vi "ImgLnExp.vi"(7 "Ln/Exp(Ln)":bool, 8 "EorIn":errorcluster, 10 "Dst":T1(plugin-control), 11 "Src":T1(plugin-control)) -> (0 "ErrOut":errorcluster, 3 "ImgOut":T1(plugin-control))   [LabVIEW 2014]
doc: "Use this template to build a VI to use as a subVI."
panel:
  out "size(s)":i32[](array[numeric])
  out "Image Pixels (Float)":sgl[][](array[numeric]) format="%.2f"
  # "Output Parameters"
  # "Input Parameters"
  # "VI Description:\nThis VI is .."
  # ":: MVi Framework V1.0 ::\nAuthor:Gaoke Yang\nEmail: gaoke.yang@yahoo.com\nWeb: www.mvicontrol.com\nCopyright (C) 2015, MVI Technologies All Rights Reserved"
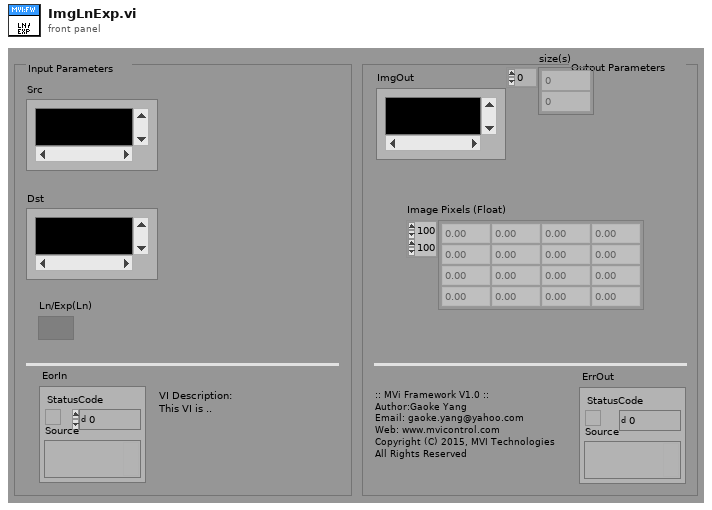
[diagram p1: front panel]
types:
  T1 = typedef "IMAQ Image.ctl" = refnum<image>
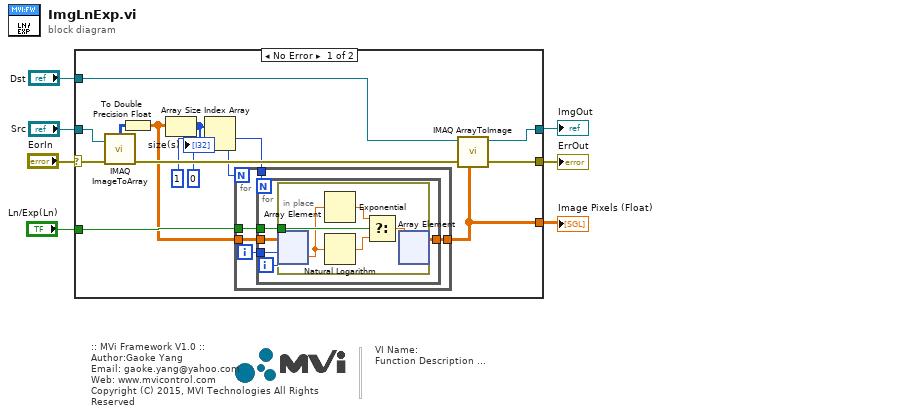
[diagram p0: block diagram]
diagram:
  # "VI Name:\nFunction Description ..."
  # ":: MVi Framework V1.0 ::\nAuthor:Gaoke Yang\nEmail: gaoke.yang@yahoo.com\nWeb: www.mvicontrol.com\nCopyright (C) 2015, MVI Technologies All Rights Reserved"
  n1 = case shown="No Error" "EorIn" {
    selector: "EorIn" -> [w22 w39]
    tunnel: [w21 w39] -> w6
    tunnel: [w18 w38] -> w4
    tunnel: "Src" -> [w19 w38]
    tunnel: "Ln/Exp(Ln)" -> [w17 _]
    tunnel: "Dst" -> [w16 _]
    tunnel: [w14 _] -> w1
    frame No Error {
      n2 = call "IMAQ ImageToArray"("error in (no error)"=w22, "Image"=w19) -> ("error out"=w20:errorcluster, "Image Pixels (U8)"=w15:u8[][])  [unwired: 2 in, 3 out]
      n3 = To Double Precision Float(number=w15) -> (double precision float=w13:dbl[][])
      n4 = Array Size(array=w13) -> (size(s)=w12:i32[])
      "size(s)" <- w12
      n5 = Index Array(array=w12, index #1=1 ("index"), index #2=0 ("index")) -> (element #1=w9:i32, element #2=w8:i32)
      n6 = for {
        N: w8 -> [_]
        tunnel: w17 -> [w27]
        tunnel: w13 -> [w25]
        tunnel: [w24] -> w14
        tunnel: w9 -> [w23]
        i -> [w26]
        n7 = for {
          N: w23 -> [_]
          tunnel: w27 -> [w30]
          tunnel: w26 -> [w31]
          tunnel: w25 -> [w29]
          tunnel: [w28] -> w24
          i -> [w32]
          n8 = in-place {
            in-place-border: w30 -> [w35]
            n9 = in-place-array #1(w29, w31, w32) -> (w34:dbl)
            n10 = Exponential(1:w34) -> (0:w37:dbl)
            n11 = Natural Logarithm(1:w34) -> (0:w36:dbl)
            n12 = Select(t=w37, s=w35, f=w36) -> (s? t:f=w33:dbl)
            n13 = in-place-array #1(w33) -> (w28:dbl[][])  [unwired: 2 out]
          }
        }
      }
      n14 = call "IMAQ ArrayToImage"("Image Pixels (Float)"=w14, "error in (no error)"=w20, "Image"=w16) -> ("error out"=w21:errorcluster, "Image Out"=w18:T1)  [unwired: 7 in]
    }
    frame Error {
    }
  }
  "ErrOut" <- w6
  "ImgOut" <- w4
  "Image Pixels (Float)" <- w1
